vi "Configure Transform Coupling.vi"(0 "VISA resource name":refnum<visa-resource-name>, 1 "Enable Transform State Coupling (F: Disable)":bool, 2 "Enable Transform Mode Coupling (T: Enable)":bool=TRUE, 5 "Channel (1)":i32=1, 9 "Enable Transform Stimulus Coupling (T: Enable)":bool=TRUE, 11 "error in (no error)":errorcluster, 12 "Enable Transform Window Coupling (T: Enable)":bool=TRUE, 13 "Enable Transform Distance Marker Units Coupling (T: Enable)":bool=TRUE) -> (4 "VISA resource name out":refnum<visa-resource-name>, 15 "error out":errorcluster)   [LabVIEW 2018, in "Keysight PNA Series.lvlib"]
doc: "Configures the time domain transform parameters to be coupled."
uses:
  Keysight PNA Series.lvlib
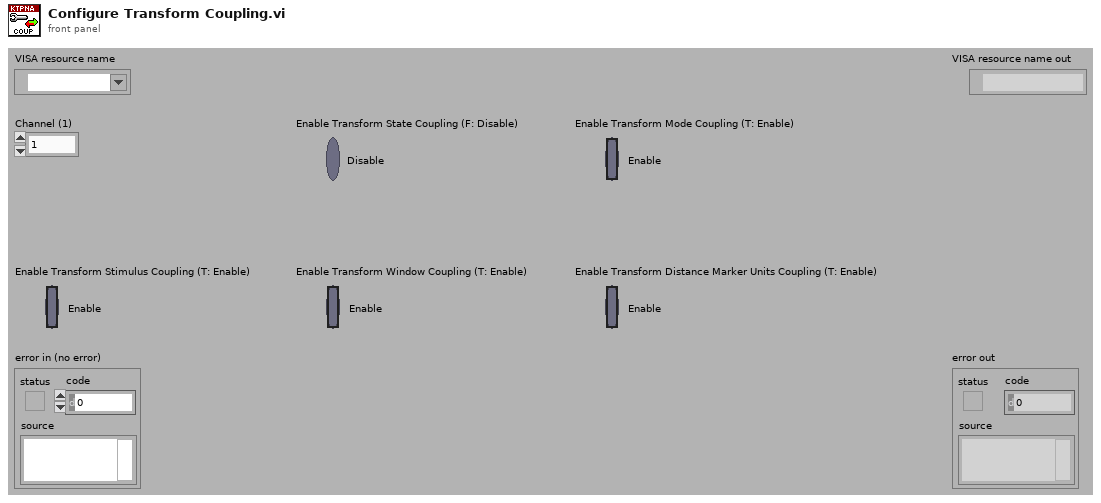
[diagram p1: front panel]
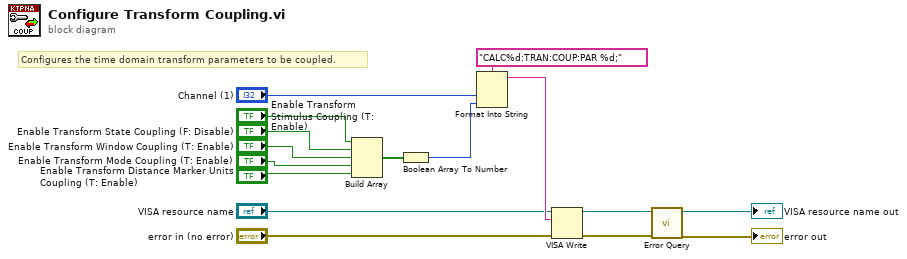
[diagram p0: block diagram]
diagram:
  # "Configures the time domain transform parameters to be coupled."
  n1 = Build Array("Enable Transform Stimulus Coupling (T: Enable)", "Enable Transform State Coupling (F: Disable)", "Enable Transform Window Coupling (T: Enable)", "Enable Transform Mode Coupling (T: Enable)", "Enable Transform Distance Marker Units Coupling (T: Enable)") -> (w2:bool[])
  n2 = Boolean Array To Number(Boolean array=w2) -> (number=w1:u32)
  n3 = Format Into String(format string="CALC%d:TRAN:COUP:PAR %d;", "Channel (1)", w1) -> (resulting string=w14:string)  [unwired: 2 in, 1 out]
  n4 = VISA Write(VISA resource name="VISA resource name", write buffer=w14, error in (no error)="error in (no error)") -> (VISA resource name out=w11:refnum<visa-resource-name>, error out=w10:errorcluster)  [unwired: 1 out]
  n5 = call "Error Query.vi"("error in (no error)"=w10, "VISA resource name"=w11) -> ("error out"=→"error out":errorcluster, "VISA resource name out"=→"VISA resource name out":refnum<visa-resource-name>)  [unwired: 6 in, 2 out]
